vi "driveForward.vi"(8 "speed (%)":dbl, 9 "distance (ft)":dbl, 10 "rightMotor":T1={"DeviceStatus"={"status"=FALSE, "code"=0, "source"=""}, "Type"=enum."PWM", "PWM"={"PWM Channel"=enum."Invalid", "DeadBand"={"Name"="", "maxPositivePwm"=0, "minPositivePwm"=0, "centerPwm"=0, "maxNegativePwm"=0, "minNegativePwm"=0, "angularRange"=0}}, "CAN"={"Device Number"=0, "SetOutput VI Ref"=variant(refnum<vi> refnum), "GetOutput VI Ref"=variant(refnum<vi> refnum), "Enable VI Ref"=variant(refnum<vi> refnum), "Disable VI Ref"=variant(refnum<vi> refnum), "Data"=variant}, "Invert"=FALSE}, 11 "leftMotor":T1={"DeviceStatus"={"status"=FALSE, "code"=0, "source"=""}, "Type"=enum."PWM", "PWM"={"PWM Channel"=enum."Invalid", "DeadBand"={"Name"="", "maxPositivePwm"=0, "minPositivePwm"=0, "centerPwm"=0, "maxNegativePwm"=0, "minNegativePwm"=0, "angularRange"=0}}, "CAN"={"Device Number"=0, "SetOutput VI Ref"=variant(refnum<vi> refnum), "GetOutput VI Ref"=variant(refnum<vi> refnum), "Enable VI Ref"=variant(refnum<vi> refnum), "Disable VI Ref"=variant(refnum<vi> refnum), "Data"=variant}, "Invert"=FALSE}) -> (2 "rightMotor":T1={"DeviceStatus"={"status"=FALSE, "code"=0, "source"=""}, "Type"=enum."PWM", "PWM"={"PWM Channel"=enum."Invalid", "DeadBand"={"Name"="", "maxPositivePwm"=0, "minPositivePwm"=0, "centerPwm"=0, "maxNegativePwm"=0, "minNegativePwm"=0, "angularRange"=0}}, "CAN"={"Device Number"=0, "SetOutput VI Ref"=variant(enum8{"Percent VBus", "Current", "Speed", "Position", "Voltage"} enum."Percent VBus"), "GetOutput VI Ref"=variant(refnum<k1> refnum), "Enable VI Ref"=variant(dbl 12.0), "Disable VI Ref"=variant(enum8{"Percent VBus", "Speed", "Position", "Slave", "Unchanged / Invalid"} enum."Percent VBus"), "Data"=variant}, "Invert"=FALSE}, 3 "leftMotor":T1={"DeviceStatus"={"status"=FALSE, "code"=0, "source"=""}, "Type"=enum."PWM", "PWM"={"PWM Channel"=enum."Invalid", "DeadBand"={"Name"="", "maxPositivePwm"=0, "minPositivePwm"=0, "centerPwm"=0, "maxNegativePwm"=0, "minNegativePwm"=0, "angularRange"=0}}, "CAN"={"Device Number"=0, "SetOutput VI Ref"=variant(enum8{"Percent VBus", "Current", "Speed", "Position", "Voltage"} enum."Percent VBus"), "GetOutput VI Ref"=variant(refnum<k1> refnum), "Enable VI Ref"=variant(dbl 12.0), "Disable VI Ref"=variant(enum8{"Percent VBus", "Speed", "Position", "Slave", "Unchanged / Invalid"} enum."Percent VBus"), "Data"=variant}, "Invert"=FALSE})   [LabVIEW 2016]
uses:
  <vilib>/Rock Robotics/WPI/MotorControl/WPI_MotorControlDeviceRef.ctl
  <vilib>/Rock Robotics/WPI/MotorControl/WPI_MotorControlType.ctl
  <vilib>/Rock Robotics/SystemInterfaces/DIO/FPGA_DIOPWMChannel.ctl
  <vilib>/Rock Robotics/WPI/PWM/WPI_PWMDeadband.ctl
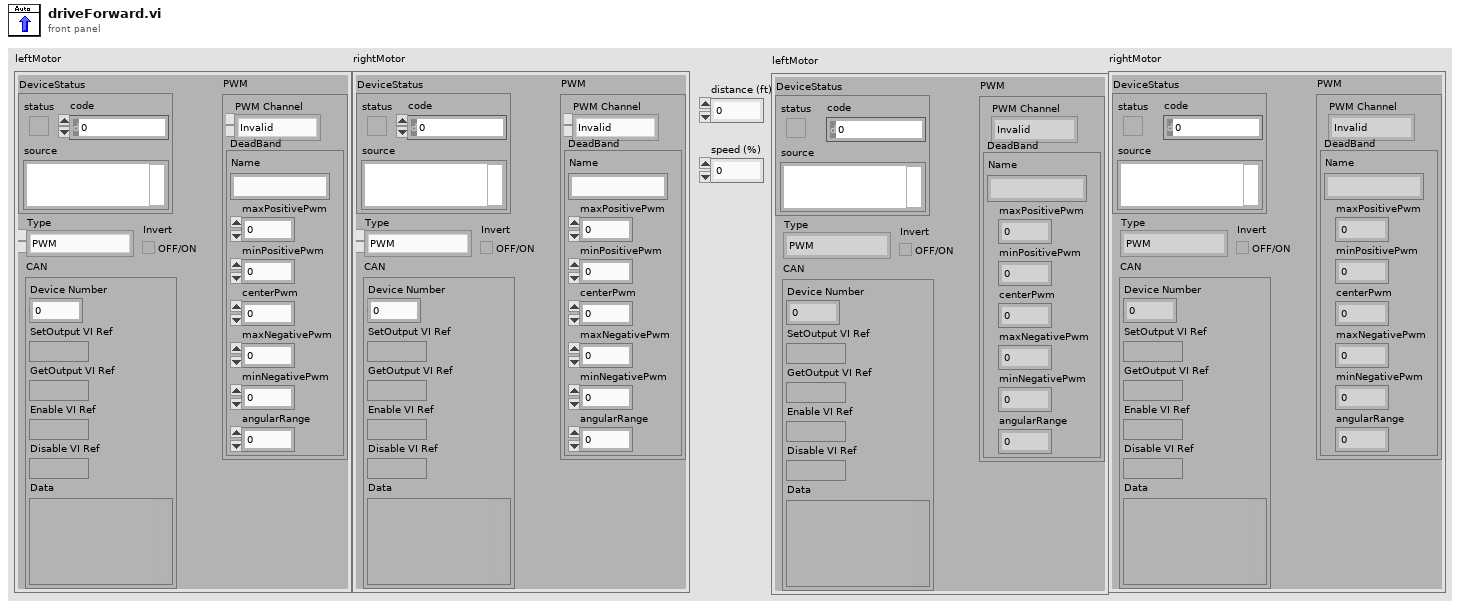
[diagram p1: front panel]
types:
  T1 = typedef "WPI_MotorControlDeviceRef.ctl" = cluster{"DeviceStatus":errorcluster, "Type":T2, "PWM":cluster{"PWM Channel":T3, "DeadBand":T4}, "CAN":cluster{"Device Number":u8, "SetOutput VI Ref":variant, "GetOutput VI Ref":variant, "Enable VI Ref":variant, "Disable VI Ref":variant, "Data":variant}, "Invert":bool}
  T2 = typedef "WPI_MotorControlType.ctl" = enum16{"PWM", "CAN"}
  T3 = typedef "FPGA_DIOPWMChannel.ctl" = enum8{"PWM 0", "PWM 1", "PWM 2", "PWM 3", "PWM 4", "PWM 5", "PWM 6", "PWM 7", "PWM 8", "PWM 9", "PWM MXP 0", "PWM MXP 1", "PWM MXP 2", "PWM MXP 3", "PWM MXP 4", "PWM MXP 5", "PWM MXP 6", "PWM MXP 7", "PWM MXP 8", "PWM MXP 9", "Invalid"}
  T4 = typedef "WPI_PWMDeadband.ctl" = cluster{"Name":string, "maxPositivePwm":i32, "minPositivePwm":i32, "centerPwm":i32, "maxNegativePwm":i32, "minNegativePwm":i32, "angularRange":u16}
  T5 = typedef "WPI_CANTalonSRX_GlobalStatus.ctl" = cluster{"Applied Throttle":dbl, "Module Enabled":bool, "CAN Error":errorcluster, "Closed Loop Error":dbl, "Forward Limit Switch Closed":bool, "Reverse Limit Switch Closed":bool, "Sensor Position":dbl, "Sensor Velocity":dbl, "Current":dbl, "Sticky Fault - Over Temp":bool, "Sticky Fault - Under Voltage":bool, "Sticky Fault - Forward Limit":bool, "Sticky Fault - Reverse Limit":bool, "Sticky Fault - Forward Soft Limit":bool, "Sticky Fault - Reverse Soft Limit":bool, "Brake is Enabled":bool, "Encoder Position":dbl, "Encoder Velocity":dbl, "Encoder Index Count":dbl, "Encoder A Pin State":bool, "Encoder B Pin State":bool, "Encoder Index Pin State":bool, "Analog In":dbl, "Analog In Velocity":dbl, "Temperature (C)":dbl, "Battery Voltage":dbl, "Control 5 Is Supported":bool, "Current Profile Slot Select":dbl, "Pos Div 8":bool, "Vel Div 4":bool, "Pulse Width Position":i32, "Pulse Width Velocity":i32, "Pulse Width Rise To Rise (us)":i32, "Pulse Width Rise To Fall (us)":i32, "Mot Prof Active Is Under Run":bool, "Mot Prof Active Has Under Run":bool, "Mot Prof Active Is Last":bool, "Mot Prof Active Velocity Only":bool, "Mot Prof Active Is Valid":bool, "Mot Prof Buffer Is Full":bool, "Mot Prof Active Profile Slot Select":i32, "Mot Prof NextID":i32, "Mot Prof Count":i32, "Mot Prof Active Velocity":dbl, "Mot Prof Active Position":dbl, "Mot Prof Output Enable":i32}
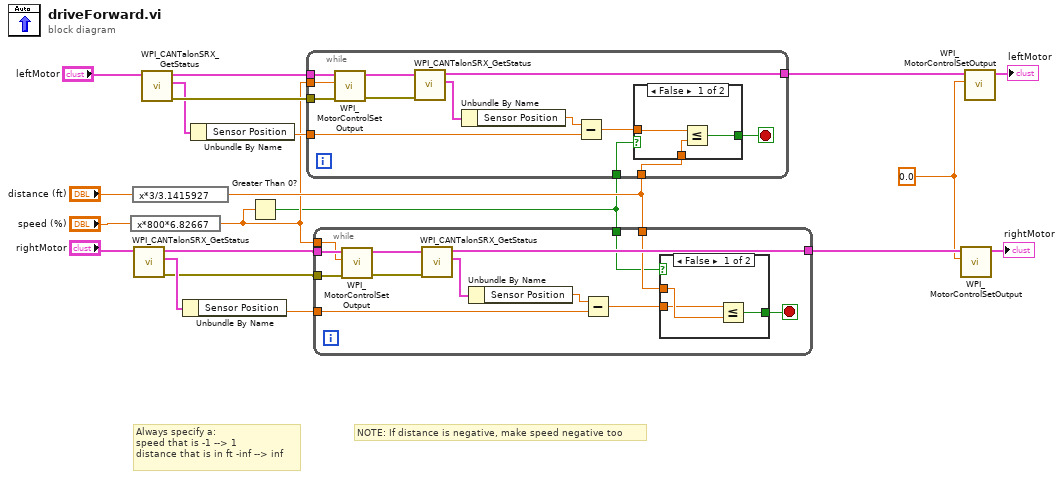
[diagram p0: block diagram]
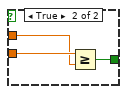
[diagram p2: hidden frame]
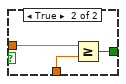
[diagram p3: hidden frame]
diagram:
  w6 = 0.0
  # "NOTE: If distance is negative, make speed negative too"
  # "Always specify a:\nspeed that is -1 --> 1\ndistance that is in ft -inf --> inf"
  n1 = expression code="x*800*6.82667"("speed (%)") -> (w2:dbl)
  n2 = expression code="x*3/3.1415927"("distance (ft)") -> (w3:dbl)
  n3 = call <vilib>:"WPI_CANTalonSRX_GetStatus.vi"("CAN Talon SRX Ref"="rightMotor") -> ("error out"=w12:errorcluster, "Talon SRX Status"=w14:T5, "CAN Talon SRX Ref"=w13:T1)  [unwired: 8 in]
  n4 = call <vilib>:"WPI_CANTalonSRX_GetStatus.vi"("CAN Talon SRX Ref"="leftMotor") -> ("error out"=w19:errorcluster, "Talon SRX Status"=w18:T5, "CAN Talon SRX Ref"=w20:T1)  [unwired: 8 in]
  n5 = Unbundle By Name(w14) -> ("Sensor Position"=w10:dbl)
  n6 = Unbundle By Name(w18) -> ("Sensor Position"=w16:dbl)
  n7 = Greater Than 0?(x=w2) -> (x > 0?=w1:bool)
  n8 = while {
    tunnel: w20 -> [w31]
    tunnel: w19 -> [w30]
    tunnel: [w28] -> w8
    tunnel: w16 -> [w26]
    tunnel: w3 -> [w23]
    tunnel: w2 -> [w24]
    tunnel: w1 -> [w22]
    stop <- w25 stop-if-true
    n9 = call <vilib>:"WPI_MotorControlSetOutput.vi"("error in (no error)"=w30, "Output"=w24, "MotorControlDevRef"=w31) -> ("error out"=w32:errorcluster, "MotorControlDevRef"=w33:T1)  [unwired: 6 in, 1 out]
    n10 = call <vilib>:"WPI_CANTalonSRX_GetStatus.vi"("error in (no error)"=w32, "CAN Talon SRX Ref"=w33) -> ("Talon SRX Status"=w29:T5, "CAN Talon SRX Ref"=w28:T1)  [unwired: 7 in, 1 out]
    n11 = Unbundle By Name(w29) -> ("Sensor Position"=w27:dbl)
    n12 = Subtract(x=w27, y=w26) -> (x-y=w21:dbl)
    n13 = case shown="False" w22 {
      tunnel: [w36 w39] -> w25
      tunnel: w21 -> [w34 w38]
      tunnel: w23 -> [w35 w37]
      frame False {
        n14 = Less Or Equal?(x=w34, y=w35) -> (x <= y?=w36:bool)
      }
      frame True {
        n15 = Greater Or Equal?(x=w38, y=w37) -> (x >= y?=w39:bool)
      }
    }
  }
  n16 = while {
    tunnel: w13 -> [w50]
    tunnel: w12 -> [w49]
    tunnel: [w47] -> w7
    tunnel: w3 -> [w42]
    tunnel: w10 -> [w44]
    tunnel: w2 -> [w43]
    tunnel: w1 -> [w41]
    stop <- w45 stop-if-true
    n17 = call <vilib>:"WPI_MotorControlSetOutput.vi"("error in (no error)"=w49, "Output"=w43, "MotorControlDevRef"=w50) -> ("error out"=w51:errorcluster, "MotorControlDevRef"=w52:T1)  [unwired: 6 in, 1 out]
    n18 = call <vilib>:"WPI_CANTalonSRX_GetStatus.vi"("error in (no error)"=w51, "CAN Talon SRX Ref"=w52) -> ("Talon SRX Status"=w48:T5, "CAN Talon SRX Ref"=w47:T1)  [unwired: 7 in, 1 out]
    n19 = Unbundle By Name(w48) -> ("Sensor Position"=w46:dbl)
    n20 = Subtract(x=w46, y=w44) -> (x-y=w40:dbl)
    n21 = case shown="False" w41 {
      tunnel: [w55 w58] -> w45
      tunnel: w40 -> [w53 w57]
      tunnel: w42 -> [w54 w56]
      frame False {
        n22 = Less Or Equal?(x=w53, y=w54) -> (x <= y?=w55:bool)
      }
      frame True {
        n23 = Greater Or Equal?(x=w57, y=w56) -> (x >= y?=w58:bool)
      }
    }
  }
  n24 = call <vilib>:"WPI_MotorControlSetOutput.vi"("Output"=w6, "MotorControlDevRef"=w7) -> ("MotorControlDevRef"=→"rightMotor":T1)  [unwired: 7 in, 2 out]
  n25 = call <vilib>:"WPI_MotorControlSetOutput.vi"("Output"=w6, "MotorControlDevRef"=w8) -> ("MotorControlDevRef"=→"leftMotor":T1)  [unwired: 7 in, 2 out]
